vi "connect.vi"(8 "error in (no error)":errorcluster, 11 "IP simple ADU in":refnum<class "SMSD ADU.lvclass">) -> (0 "error out":errorcluster, 3 "IP simple ADU out":refnum<class "SMSD ADU.lvclass">)   [LabVIEW 2021, in "SMSD ADU.lvclass"]
doc: "Opens a TCP connection to the address and port stored in the class."
uses:
  SMSD ADU.lvclass
  SMSD ADU.lvclass/SMSD ADU.ctl
  <vilib>/Utility/error.llb/Clear Errors.vi
  Modbus_v121c/Network Interface/TCP Interface/TSC/TCP Shared Components.lvlib
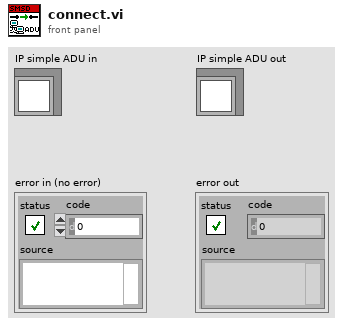
[diagram p1: front panel]
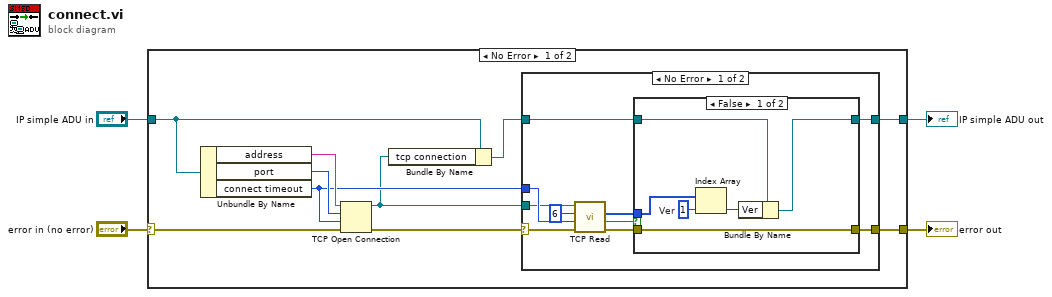
[diagram p0: block diagram]
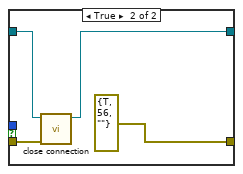
[diagram p2: hidden frame]
diagram:
  n1 = case shown="No Error" "error in (no error)" {
    selector: "error in (no error)" -> [w11 w37]
    tunnel: [w10 w37] -> w4
    tunnel: "IP simple ADU in" -> [w12 w38]
    tunnel: [w5 w38] -> w2
    frame No Error {
      n2 = Unbundle By Name(w12) -> ("address"=w14:string, "port"=w13:u16, "connect timeout"=w9:i32)
      n3 = TCP Open Connection(address=w14, remote port or service name=w13, timeout ms (60000)=w9, error in (no error)=w11) -> (connection ID=w8:refnum<k5>, error out=w7:errorcluster)  [unwired: 1 in]
      n4 = Bundle By Name(cluster=w12, "tcp connection"=w8) -> (w6:refnum<class "SMSD ADU.lvclass">)
      n5 = case shown="No Error" w7 {
        selector: w7 -> [w20 w35]
        tunnel: [w15 w35] -> w10
        tunnel: w9 -> [w23 _]
        tunnel: w8 -> [w21 _]
        tunnel: w6 -> [w18 w36]
        tunnel: [w19 w36] -> w5
        frame No Error {
          n6 = call "TCP Read.vi"("error in"=w20, "timeout"=w23, "bytes to read"=6, "connection ID"=w21) -> ("error out"=w17:errorcluster, "timed out?"=w16:bool, "data"=w22:u8[])  [unwired: 4 in, 1 out]
          n7 = case shown="False" w16 {
            tunnel: w22 -> [w28 _]
            tunnel: [w27 w32] -> w19
            tunnel: w18 -> [w26 w34]
            tunnel: w17 -> [w25 w33]
            tunnel: [w25 errorcluster {"status"=TRUE, "code"=56, "source"=""} ("error IO")] -> w15
            frame False {
              w30 = 1  # Ver
              n8 = Index Array(array=w28, index=w30) -> (element=w29:u8)
              n9 = Bundle By Name(cluster=w26, "Ver"=w29) -> (w27:refnum<class "SMSD ADU.lvclass">)
            }
            frame True {
              n10 = call "close connection.vi"("error in"=w33, "TCP master in"=w34) -> ("TCP master out"=w32:refnum<class "SMSD ADU.lvclass">)  [unwired: 8 in, 1 out]
            }
          }
        }
        frame Error {
        }
      }
    }
    frame Error {
    }
  }
  "error out" <- w4
  "IP simple ADU out" <- w2
